vi "user initialization.vi"(8 "error in":errorcluster, 10 "configuration in":refnum<class "control module configuration.lvclass">, 11 "Temperature Chamber Model runtime in":refnum<class "Temperature Chamber Model runtime.lvclass">) -> (0 "error out":errorcluster, 3 "Temperature Chamber Model runtime out":refnum<class "Temperature Chamber Model runtime.lvclass">)   [LabVIEW 2013, in "Temperature Chamber Model runtime.lvclass"]
uses:
  Temperature Chamber Model runtime.lvclass
  <vilib>/NI/DCAF/Tag Editor Core/control module/configuration/control module configuration.lvclass
  configuration/Temperature Chamber Model configuration.lvclass
  <vilib>/NI/DCAF/Tag Editor Core/control module/runtime/control module runtime.lvclass
  Temperature Chamber Model runtime.lvclass/Temperature Chamber Model runtime.ctl
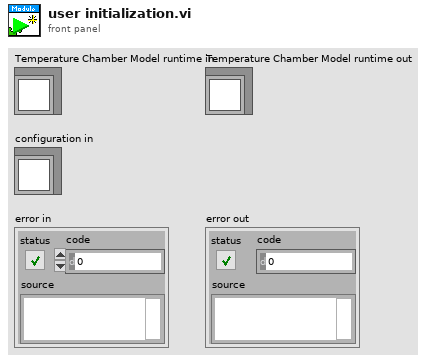
[diagram p1: front panel]
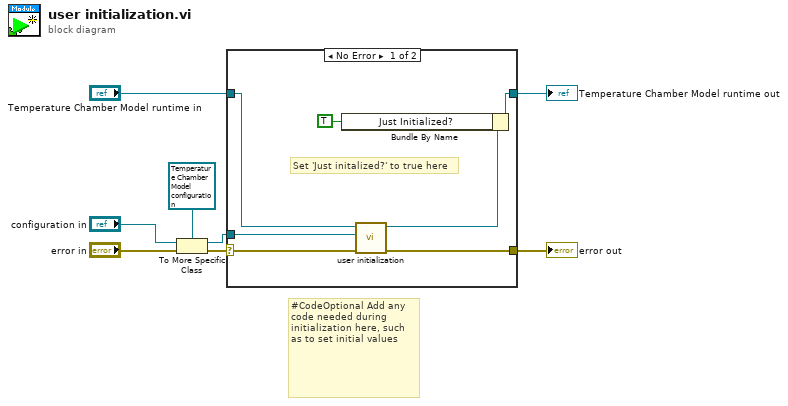
[diagram p0: block diagram]
diagram:
  # "#CodeOptional Add any code needed during initialization here, such as to set initial values"
  n1 = To More Specific Class(target class=refnum<class "Temperature Chamber Model configuration.lvclass"> refnum ("user module configuration"), reference="configuration in", error in="error in") -> (specific class reference=w1:refnum<class "Temperature Chamber Model configuration.lvclass">, error out=w5:errorcluster)
  n2 = case shown="No Error" w5 {
    selector: w5 -> [w15 w16]
    tunnel: [w14 w17] -> w4
    tunnel: "Temperature Chamber Model runtime in" -> [w11 w17]
    tunnel: [w12 w16] -> w2
    tunnel: w1 -> [w9 _]
    frame No Error {
      # "Set 'Just initalized?' to true here"
      n3 = call-parent "user initialization.vi"("error in"=w15, "configuration in"=w9, "fixed channel runtime in"=w11) -> ("error out"=w12:errorcluster, "fixed channel runtime out"=w10:refnum<class "Temperature Chamber Model runtime.lvclass">)  [unwired: 7 in]
      n4 = Bundle By Name(cluster=w10, "Just Initialized?"=TRUE ("Model State.Just Initialized?")) -> (w14:refnum<class "Temperature Chamber Model runtime.lvclass">)
    }
    frame Error {
    }
  }
  "error out" <- w2
  "Temperature Chamber Model runtime out" <- w4
